vi "IR120917 Transmission ref av elec_SD.vi"(1 "resultat_input":dbl[](array[numeric])=array[24576 elements]) -> (0 "Résultat Transmission":dbl[][](array[numeric]))   [LabVIEW 2015]
uses:
  globalVarSD.vi
panel:
  out "Out":dbl[][](graph)
  out "In":dbl[](graph)
  # "Transmission: on fait le log après la moyenne.\n\nCe VI comporte une entrée Dark: dark shutter fermé. La laisser à 0 \nce dark doit être retiré à toute les données, puis on doit faire le meme calcul avec le reste de Idark -dark à la place de Idark.s"
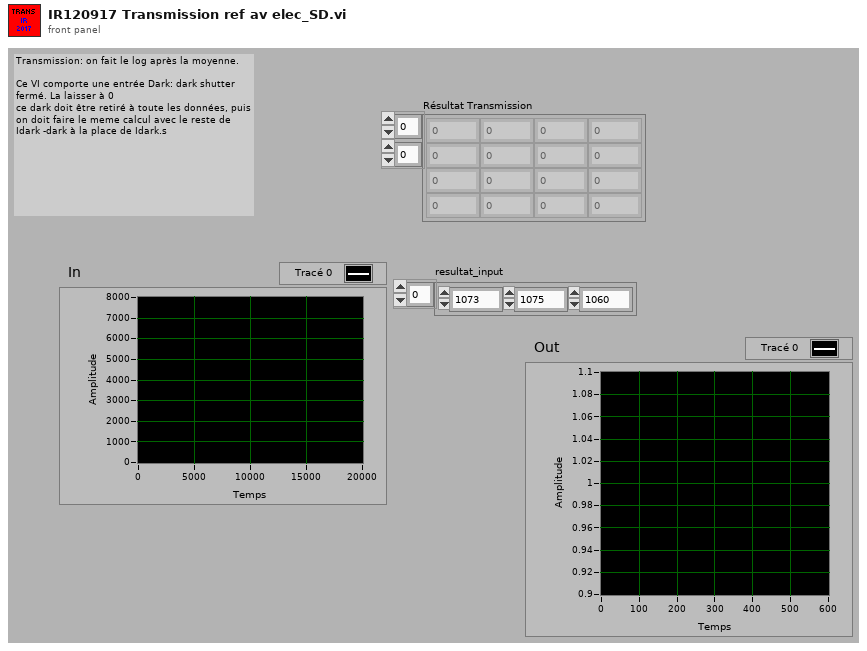
[diagram p1: front panel]
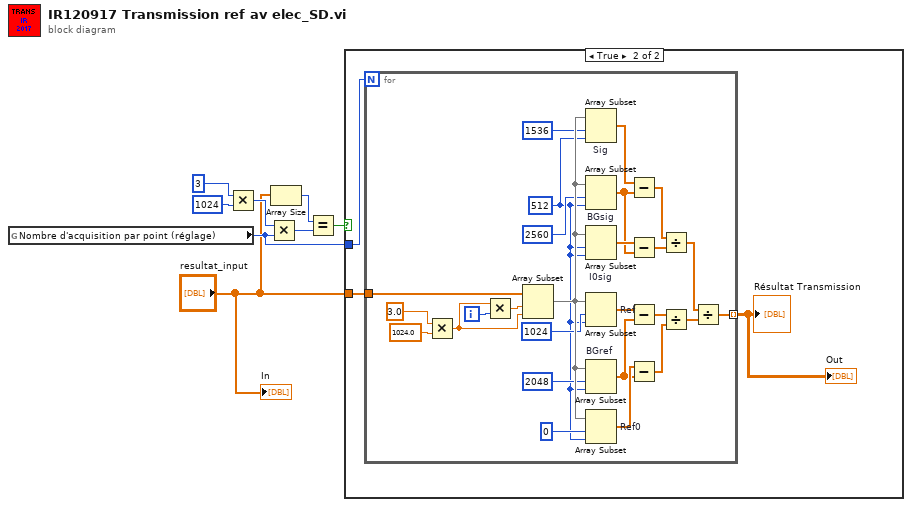
[diagram p0: block diagram]
diagram:
  n1 = global read "globalVarSD.vi" "Nombre d'acquisition par point (réglage)"() -> (w2:u32)
  n2 = Multiply(x=3, y=1024) -> (x*y=w6:i32)
  n3 = Multiply(x=w6, y=w2) -> (x*y=w4:u32)
  n4 = Array Size(array="resultat_input") -> (size(s)=w5:i32)
  n5 = Equal?(x=w5, y=w4) -> (x = y?=w3:bool)
  n6 = case shown="True" w3 {
    tunnel: "resultat_input" -> [_ w11]
    tunnel: w2 -> [_ w10]
    frame False {
    }
    frame True {
      n7 = for {
        N: w10 -> [_]
        tunnel: w11 -> [w35]
        tunnel: [w13] -> w9 mode=indexing
        i -> [w19]
        w12 = 512 ("longueur")
        n8 = Multiply(x=3.0, y=1024.0) -> (x*y=w33:dbl)
        n9 = Multiply(x=w33, y=w19) -> (x*y=w34:dbl)
        n10 = Array Subset(array=w35, index=w34, length=w33) -> (w22:dbl[])
        n11 = Array Subset "Sig"(array=w22, index=1536 ("indice"), length=w12) -> (w31:dbl[])
        n12 = Array Subset "BGsig"(array=w22, index=2560 ("indice"), length=w12) -> (w17:dbl[])
        n13 = Array Subset "I0sig"(array=w22, index=w12, length=w12) -> (w29:dbl[])
        n14 = Array Subset "Ref"(array=w22, index=1024 ("indice"), length=w12) -> (w32:dbl[])
        n15 = Array Subset "BGref"(array=w22, index=2048 ("indice"), length=w12) -> (w18:dbl[])
        n16 = Array Subset "Ref0"(array=w22, index=0 ("indice"), length=w12) -> (w30:dbl[])
        n17 = Subtract(x=w31, y=w17) -> (x-y=w28:dbl[])
        n18 = Subtract(x=w29, y=w17) -> (x-y=w27:dbl[])
        n19 = Subtract(x=w32, y=w18) -> (x-y=w26:dbl[])
        n20 = Subtract(x=w30, y=w18) -> (x-y=w25:dbl[])
        n21 = Divide(x=w28, y=w27) -> (x/y=w24:dbl[])
        n22 = Divide(x=w26, y=w25) -> (x/y=w23:dbl[])
        n23 = Divide(x=w24, y=w23) -> (x/y=w13:dbl[])
      }
      "Résultat Transmission" <- w9
      "Out" <- w9
    }
  }
  "In" <- "resultat_input"
